vi "plot state machine 1.vi"(0 "current":dbl, 1 "t0":dbl, 5 "Voltage":dbl, 7 "Voltage target":dbl, 11 "error in":errorcluster, 12 "Enum":enum16{"Reset", "Plot"}(ring)) -> (4 "Current plot":T1, 6 "Voltage plot":cluster{"t0":dbl, "dt":dbl, dbl[][]}, 14 "dt":dbl, 15 "error out":errorcluster)   [LabVIEW 2020]
panel:
  out "counts":i32
  out "relative seconds":dbl format="%_19f"
  out "target array":dbl[](array[numeric])
  out "Voltage array":dbl[](array[numeric])
  out "Current array":dbl[](array[numeric])
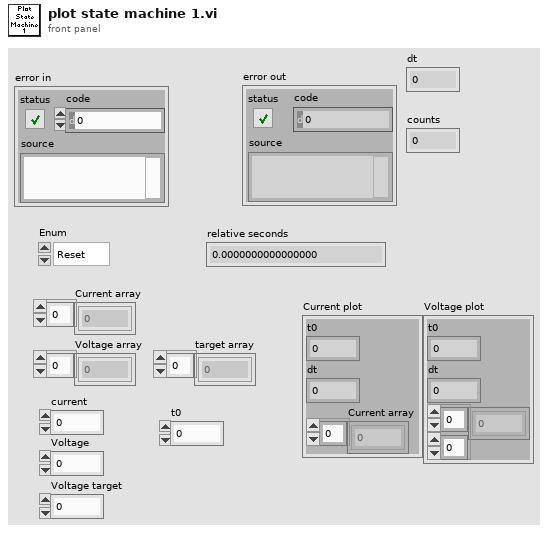
[diagram p1: front panel]
types:
  T1 = cluster{"t0":dbl, "dt":dbl, "Current array":dbl[]}
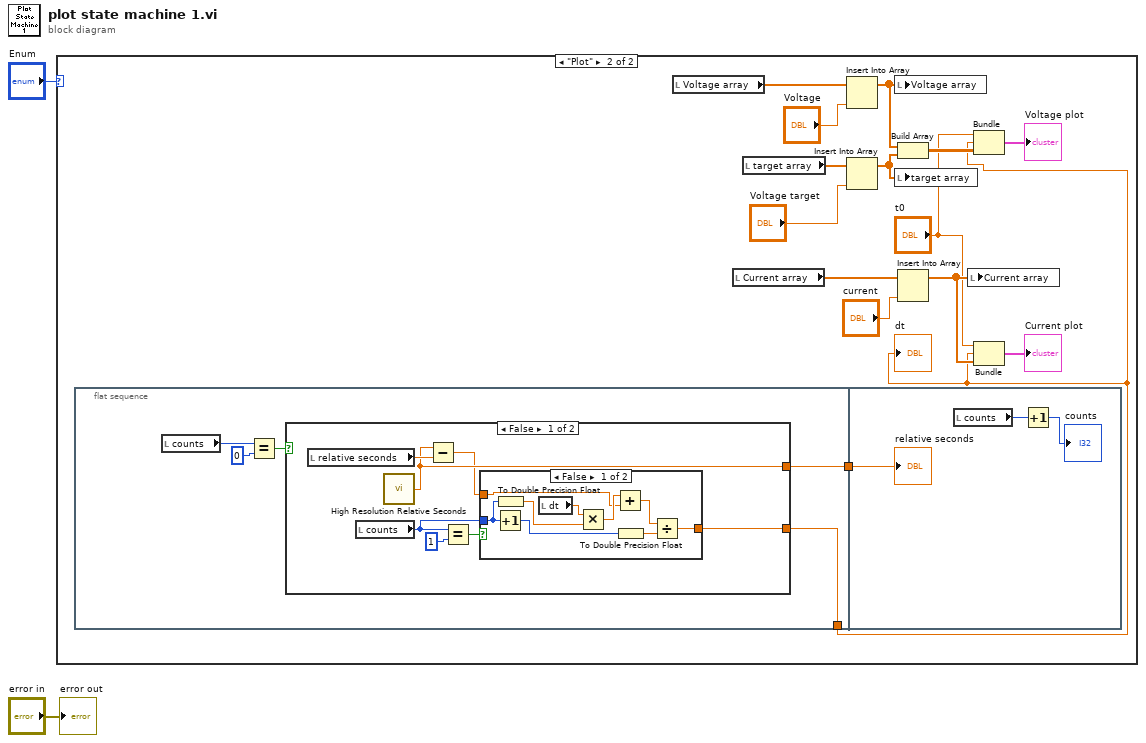
[diagram p0: block diagram]
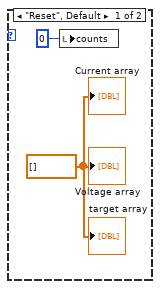
[diagram p2: hidden frame]
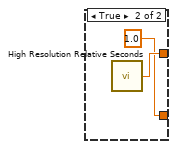
[diagram p4: hidden frame]
diagram:
  n1 = case shown="\"Plot\"" "Enum" {
    frame "Reset", Default {
      w4 = dbl[] []
      n2 = local write "counts"(0 ("counts")) -> ()
      "Current array" <- w4
      "Voltage array" <- w4
      "target array" <- w4
    }
    frame "Plot" {
      n3 = flat-sequence {
        tunnel: [w21] -> w6
        tunnel: [w20] -> w5
        tunnel: w6 -> [w46]
        frame #0 {
          n4 = local read "counts"() -> (w24:i32)
          n5 = Equal?(x=w24, y=0) -> (x = y?=w22:bool)
          n6 = case shown="False" w22 {
            tunnel: [w30 w43] -> w21
            tunnel: [w26 1.0] -> w20
            frame False {
              n7 = local read "relative seconds"() -> (w31:dbl)
              n8 = local read "counts"() -> (w25:i32)
              n9 = call <vilib>:"High Resolution Relative Seconds.vi"() -> ("relative seconds"=w30:dbl)
              n10 = Subtract(x=w30, y=w31) -> (x-y=w27:dbl)
              n11 = Equal?(x=w25, y=1) -> (x = y?=w28:bool)
              n12 = case shown="False" w28 {
                tunnel: [w32 w41] -> w26
                tunnel: w27 -> [w37 w41]
                tunnel: w25 -> [w34 _]
                frame False {
                  n13 = Increment(x=w34) -> (x+1=w35:i32)
                  n14 = To Double Precision Float(number=w34) -> (double precision float=w39:dbl)
                  n15 = local read "dt"() -> (w40:dbl)
                  n16 = Multiply(x=w40, y=w39) -> (x*y=w38:dbl)
                  n17 = Add(x=w38, y=w37) -> (x+y=w36:dbl)
                  n18 = To Double Precision Float(number=w35) -> (double precision float=w33:dbl)
                  n19 = Divide(x=w36, y=w33) -> (x/y=w32:dbl)
                }
                frame True {
                }
              }
            }
            frame True {
              n20 = call <vilib>:"High Resolution Relative Seconds.vi"() -> ("relative seconds"=w43:dbl)
            }
          }
        }
        frame #1 {
          n21 = local read "counts"() -> (w45:i32)
          n22 = Increment(x=w45) -> (x+1=→"counts":i32)
          "relative seconds" <- w46
        }
      }
      n23 = local read "Voltage array"() -> (w16:dbl[])
      n24 = local read "Current array"() -> (w19:dbl[])
      n25 = local read "target array"() -> (w14:dbl[])
      n26 = Insert Into Array(array=w16, new element="Voltage") -> (w11:dbl[])  [unwired: 1 in]
      n27 = Insert Into Array(array=w14, new element="Voltage target") -> (w10:dbl[])  [unwired: 1 in]
      n28 = local write "Voltage array"(w11) -> ()
      n29 = local write "target array"(w10) -> ()
      n30 = Build Array(w11, w10) -> (w9:dbl[][])
      n31 = Insert Into Array(array=w19, new element="current") -> (w13:dbl[])  [unwired: 1 in]
      n32 = local write "Current array"(w13) -> ()
      n33 = Bundle("t0"="t0", w5, w9) -> (→"Voltage plot":cluster{"t0":dbl, dbl, dbl[][]})  [unwired: 1 in]
      n34 = Bundle("t0"="t0", w5, "Current array"=w13) -> (→"Current plot":cluster{"t0":dbl, dbl, "Current array":dbl[]})  [unwired: 1 in]
      "dt" <- w5
    }
  }
  "error out" <- "error in"
